vi "Filter Class Tree_MAIN.vi"(9 "Show":T2={"Show Private"=TRUE, "Show Scripting"=FALSE}, 10 "Filter":string, 11 "Class Items In":T3[](array[typedef])) -> (0 "Indents OK":bool, 1 "Disabled?":bool[](array[boolean]), 2 "Class Tree Arr":T1(array[cluster]))   [LabVIEW 2023]
uses:
  class/Class Item Cluster.ctl
panel:
  out "Out size":i32
  out "In Size":i32
  out "Class Items Out Filtered":T3[](array[typedef])
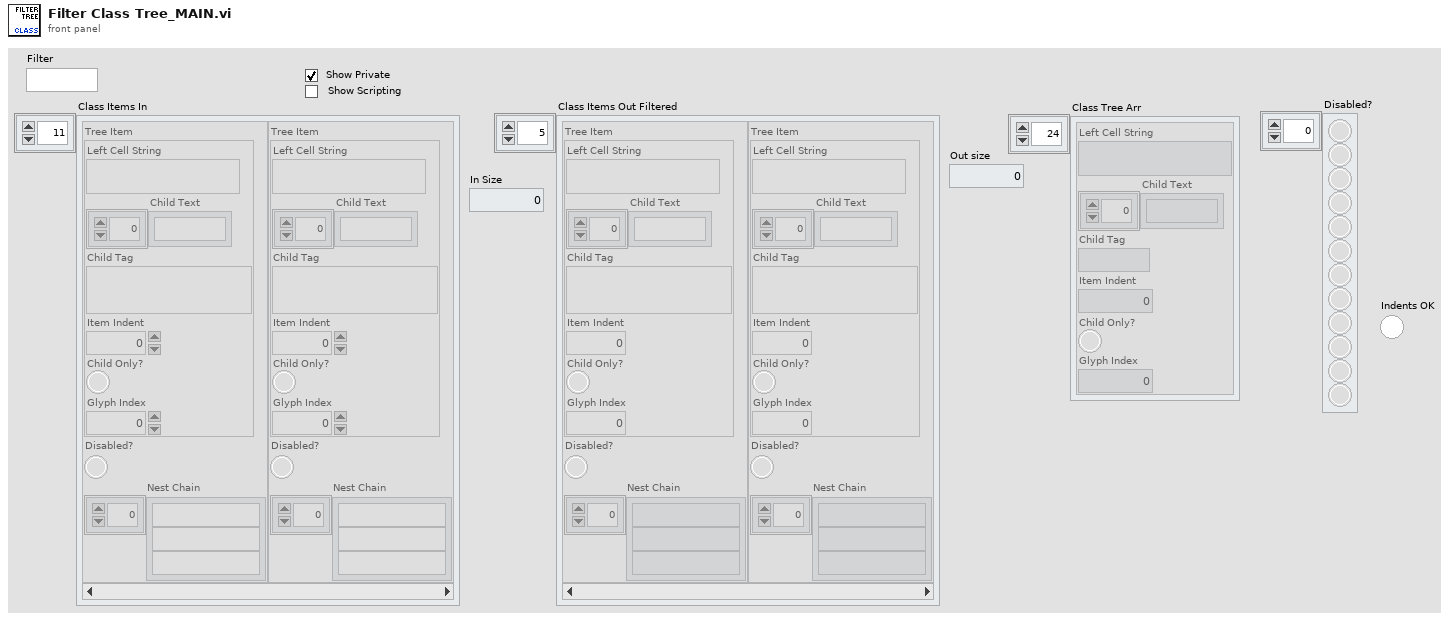
[diagram p1: front panel]
types:
  T1 = cluster{"Left Cell String":string, "Child Text":string[], "Child Tag":string, "Item Indent":i32, "Child Only?":bool, "Glyph Index":i32}[]
  T2 = cluster{"Show Private":bool, "Show Scripting":bool}
  T3 = typedef "Class Item Cluster.ctl" = cluster{"Tree Item":cluster{"Left Cell String":string, "Child Text":string[], "Child Tag":string, "Item Indent":i32, "Child Only?":bool, "Glyph Index":i32}, "Disabled?":bool, "Nest Chain":string[]}
  T4 = cluster{"Left Cell String":string, "Child Text":string[], "Child Tag":string, "Item Indent":i32, "Child Only?":bool, "Glyph Index":i32}
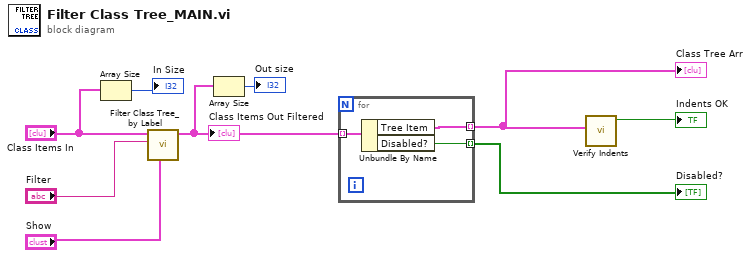
[diagram p0: block diagram]
diagram:
  n1 = Array Size(array="Class Items In") -> (size(s)=→"In Size":i32)
  n2 = call "Filter Class Tree_by Label.vi"("Show"="Show", "Filter Str"="Filter", "Class Tree Array"="Class Items In") -> ("Class Tree Array"=w4:T3[])  [unwired: 8 in]
  "Class Items Out Filtered" <- w4
  n3 = Array Size(array=w4) -> (size(s)=→"Out size":i32)
  n4 = for {
    tunnel: w4 -> [w12] mode=indexing
    tunnel: [w11] -> w6 mode=indexing
    tunnel: [w10] -> w5 mode=indexing
    n5 = Unbundle By Name(w12) -> ("Tree Item"=w11:T4, "Disabled?"=w10:bool)
  }
  "Disabled?" <- w5
  "Class Tree Arr" <- w6
  n6 = call "Verify Indents.vi"("Tree Arr"=w6) -> ("Indents OK"=→"Indents OK":bool)  [unwired: 9 in, 1 out]
